vi "Log Error.vi"(8 "error in (no error)":errorcluster, 10 "Error":string, 11 "Mag Lab Error Handler in":refnum<class "Mag Lab Error Handler.lvclass">) -> (0 "error out":errorcluster, 3 "Mag Lab Error Handler out":refnum<class "Mag Lab Error Handler.lvclass">)   [LabVIEW 2015, in "Mag Lab Error Handler.lvlib" / "Mag Lab Error Handler.lvclass"]
uses:
  Mag Lab Error Handler.lvclass
  Mag Lab Error Handler.lvclass/Mag Lab Error Handler.ctl
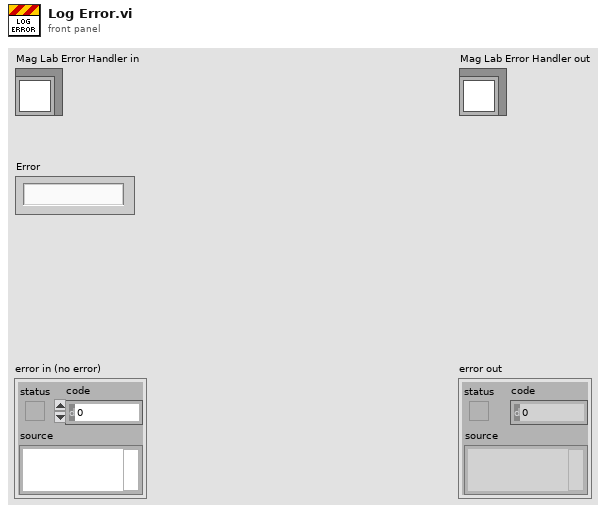
[diagram p1: front panel]
types:
  T1 = enum16{"open", "replace", "create", "open or create", "replace or create", "replace or create with confirmation"}
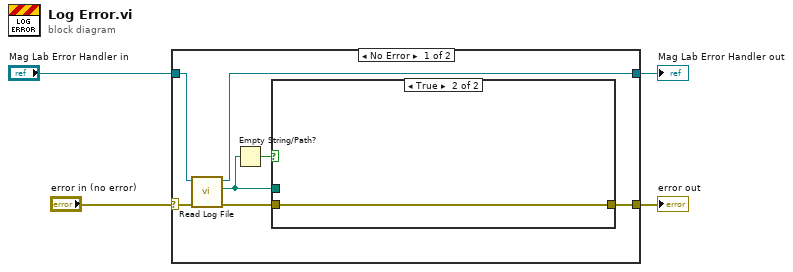
[diagram p0: block diagram]
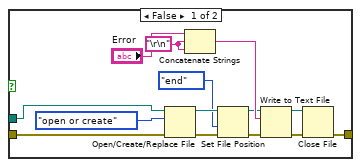
[diagram p2: hidden frame]
diagram:
  n1 = case shown="No Error" "error in (no error)" {
    selector: "error in (no error)" -> [w7 w28]
    tunnel: [w5 w28] -> w3
    tunnel: [w8 w27] -> w1
    tunnel: "Mag Lab Error Handler in" -> [w9 w27]
    frame No Error {
      n2 = call "Read Log File.vi"("error in (no error)"=w7, "Mag Lab Error Handler in"=w9) -> ("error out"=w6:errorcluster, "Log File"=w10:path, "Mag Lab Error Handler out"=w8:refnum<class "Mag Lab Error Handler.lvclass">)  [unwired: 7 in]
      n3 = Empty String/Path?(string/path=w10) -> (empty?=w11:bool)
      n4 = case shown="True" w11 {
        tunnel: w10 -> [w25 _]
        tunnel: w6 -> [w13 w26]
        tunnel: [w12 w26] -> w5
        frame False {
          w23 = "\r\n"
          n5 = Open/Create/Replace File(file path (use dialog)=w25, error in=w13, operation (0:open)=T1."open or create") -> (refnum out=w22:refnum<file>, error out=w18:errorcluster)  [unwired: 3 in, 1 out]
          n6 = Concatenate Strings("Error", w23, w23) -> (w24:string)
          n7 = Set File Position(refnum=w22, from (0:start)=enum16{"start", "end", "current"}."end", error in=w18) -> (refnum out=w20:refnum<file>, error out=w17:errorcluster)  [unwired: 1 in]
          n8 = Write to Text File(file (use dialog)=w20, text=w24, error in=w17) -> (refnum out=w15:refnum<file>, error out=w16:errorcluster)  [unwired: 1 in, 1 out]
          n9 = Close File(refnum=w15, error in=w16) -> (error out=w12:errorcluster)  [unwired: 1 out]
        }
        frame True {
        }
      }
    }
    frame Error {
    }
  }
  "error out" <- w3
  "Mag Lab Error Handler out" <- w1
